vi "Create PVConnections.vi"(8 "error in (no error)":errorcluster, 11 "BNT_ULx-MCSV in":refnum<class "BNT_ULx-MCSV.lvclass">) -> (0 "error out":errorcluster, 3 "BNT_ULx-MCSV out":refnum<class "BNT_ULx-MCSV.lvclass">)   [LabVIEW 2021, in "BNT_ULx.lvlib" / "BNT_ULx-MCSV.lvclass"]
doc: "Create PVConnection objects"
uses:
  BNT_ULx-MCSV.lvclass
  C:/Users/Holger/Documents/LVP/CSPP/CSPP-Template/Packages/CSPP_Core/Actors/CSPP_BaseActor/CSPP_BaseActor.lvclass
  CSPP_Core/Actors/CSPP_BaseActor/CSPP_BaseActor.lvclass/CSPP_BaseActor.ctl
  BNT_ULx-MCSV.lvclass/BNT_ULx-MCSV.ctl
  CSPP_Core/Classes/CSPP_BaseClasses/Factory/CSPP_Factory.lvclass
  CSPP_Core/Actors/CSPP_BaseActor/CSPP_BaseActor.lvclass
  CSPP_Core/Classes/CSPP_ProcessVariables/CSPP_ProcessVariables.lvlib
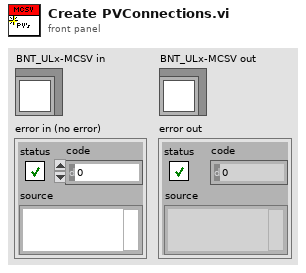
[diagram p1: front panel]
types:
  T1 = cluster{string, "Type Descriptor":string, string}
  T2 = cluster{"initial string":string, "Type Descriptor":string, string}
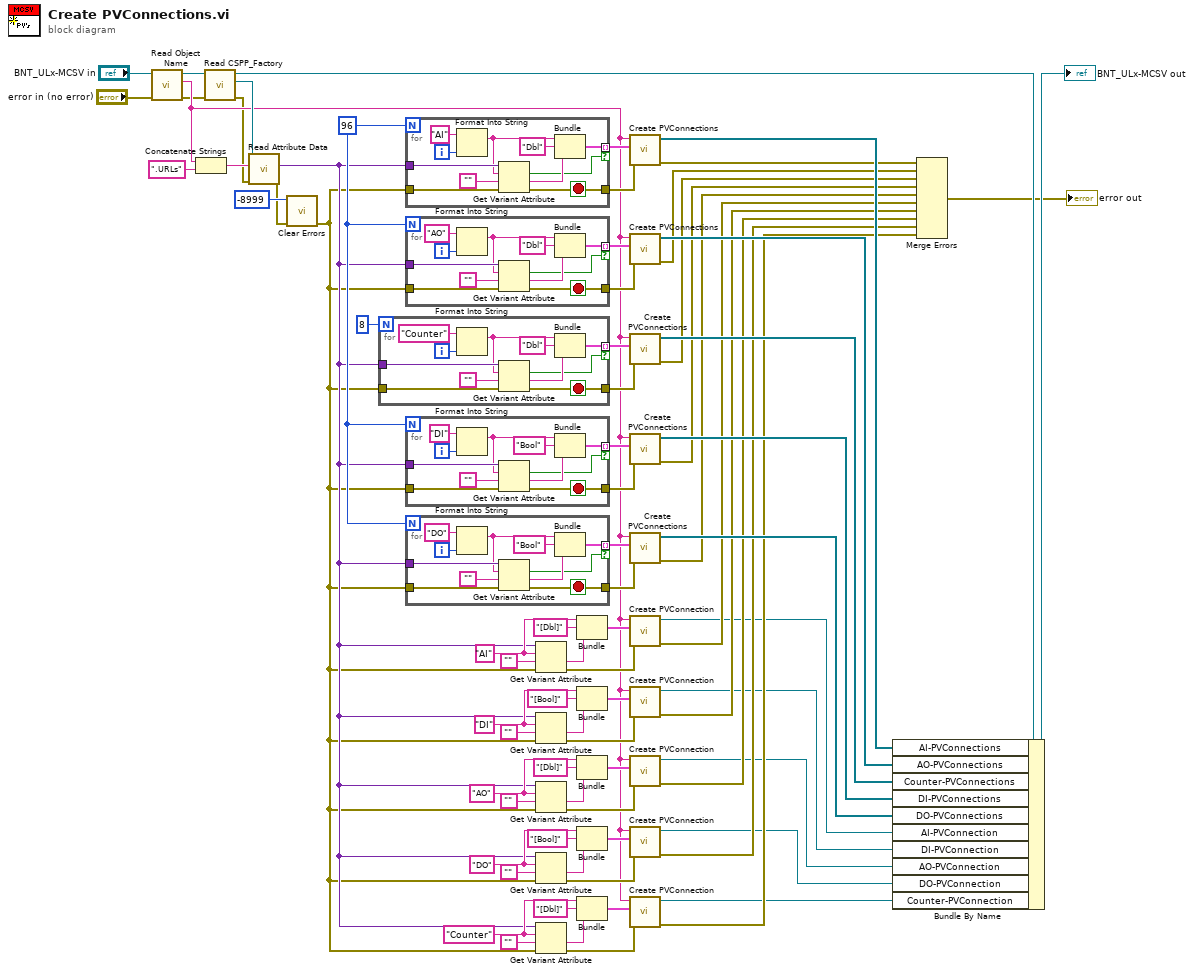
[diagram p0: block diagram]
diagram:
  w20 = "Counter" ("initial string")
  w34 = "DO" ("initial string")
  w27 = "AO" ("initial string")
  w40 = "DI" ("initial string")
  w48 = "AI" ("initial string")
  w52 = 96
  n1 = call "Read Object Name.vi"("error in (no error)"="error in (no error)", "CSPP_BaseActor in"="BNT_ULx-MCSV in") -> ("error out"=w4:errorcluster, "Object Name"=w16:string, "CSPP_BaseActor out"=w78:refnum<class "BNT_ULx-MCSV.lvclass">)  [unwired: 7 in]
  n2 = Concatenate Strings(w16, ".URLs" ("string")) -> (w76:string)
  n3 = call "Read CSPP_Factory.vi"("error in (no error)"=w4, "CSPP_BaseActor in"=w78) -> ("error out"=w3:errorcluster, "CSPP_Factory"=w73:refnum<class "CSPP_Factory.lvclass">, "CSPP_BaseActor out"=w7:refnum<class "BNT_ULx-MCSV.lvclass">)  [unwired: 7 in]
  n4 = call-dynamic "Read Attribute Data.vi"("error in (no error)"=w3, "Object Name"=w76, "CSPP_Factory in"=w73) -> ("error out"=w74:errorcluster, "Attribute Data"=w15:variant)  [unwired: 6 in, 1 out]
  n5 = call <vilib>:"Clear Errors.vi"("error in (no error)"=w74, "specific error code to clear (0: all)"=-8999) -> ("error out"=w14:errorcluster)  [unwired: 4 in, 1 out]
  n6 = for {
    N: 8 -> [_]
    tunnel: w15 -> [w88]
    tunnel: w14 -> [w87]
    tunnel: [w83] -> w63 mode=indexing if=w80
    tunnel: [w79] -> w62
    i -> [w86]
    stop <- w79 stop-if-true
    n7 = Format Into String(initial string="Counter", w86) -> (resulting string=w84:string)  [unwired: 2 in, 1 out]
    n8 = Get Variant Attribute(Variant=w88, name=w84, default value (empty Variant)="", error in=w87) -> (found=w80:bool, value=w81:string, error out=w79:errorcluster)  [unwired: 1 out]
    n9 = Bundle(w84, "Type Descriptor"="Dbl", w81) -> (w83:T1)  [unwired: 1 in]
  }
  n10 = for {
    N: w52 -> [_]
    tunnel: w15 -> [w99]
    tunnel: w14 -> [w98]
    tunnel: [w94] -> w71 mode=indexing if=w91
    tunnel: [w90] -> w68
    i -> [w97]
    stop <- w90 stop-if-true
    n11 = Format Into String(initial string="AI", w97) -> (resulting string=w95:string)  [unwired: 2 in, 1 out]
    n12 = Get Variant Attribute(Variant=w99, name=w95, default value (empty Variant)="", error in=w98) -> (found=w91:bool, value=w92:string, error out=w90:errorcluster)  [unwired: 1 out]
    n13 = Bundle(w95, "Type Descriptor"="Dbl", w92) -> (w94:T1)  [unwired: 1 in]
  }
  n14 = for {
    N: w52 -> [_]
    tunnel: w15 -> [w110]
    tunnel: w14 -> [w109]
    tunnel: [w105] -> w66 mode=indexing if=w102
    tunnel: [w101] -> w67
    i -> [w108]
    stop <- w101 stop-if-true
    n15 = Format Into String(initial string="AO", w108) -> (resulting string=w106:string)  [unwired: 2 in, 1 out]
    n16 = Get Variant Attribute(Variant=w110, name=w106, default value (empty Variant)="", error in=w109) -> (found=w102:bool, value=w103:string, error out=w101:errorcluster)  [unwired: 1 out]
    n17 = Bundle(w106, "Type Descriptor"="Dbl", w103) -> (w105:T1)  [unwired: 1 in]
  }
  n18 = for {
    N: w52 -> [_]
    tunnel: w15 -> [w121]
    tunnel: w14 -> [w120]
    tunnel: [w116] -> w58 mode=indexing if=w113
    tunnel: [w112] -> w57
    i -> [w119]
    stop <- w112 stop-if-true
    n19 = Format Into String(initial string="DI", w119) -> (resulting string=w117:string)  [unwired: 2 in, 1 out]
    n20 = Get Variant Attribute(Variant=w121, name=w117, default value (empty Variant)="", error in=w120) -> (found=w113:bool, value=w114:string, error out=w112:errorcluster)  [unwired: 1 out]
    n21 = Bundle(w117, "Type Descriptor"="Bool", w114) -> (w116:T1)  [unwired: 1 in]
  }
  n22 = for {
    N: w52 -> [_]
    tunnel: w15 -> [w132]
    tunnel: w14 -> [w131]
    tunnel: [w127] -> w53 mode=indexing if=w124
    tunnel: [w123] -> w54
    i -> [w130]
    stop <- w123 stop-if-true
    n23 = Format Into String(initial string="DO", w130) -> (resulting string=w128:string)  [unwired: 2 in, 1 out]
    n24 = Get Variant Attribute(Variant=w132, name=w128, default value (empty Variant)="", error in=w131) -> (found=w124:bool, value=w125:string, error out=w123:errorcluster)  [unwired: 1 out]
    n25 = Bundle(w128, "Type Descriptor"="Bool", w125) -> (w127:T1)  [unwired: 1 in]
  }
  n26 = Get Variant Attribute(Variant=w15, name=w48, default value (empty Variant)="", error in=w14) -> (value=w47:string, error out=w44:errorcluster)  [unwired: 2 out]
  n27 = Get Variant Attribute(Variant=w15, name=w40, default value (empty Variant)="", error in=w14) -> (value=w41:string, error out=w43:errorcluster)  [unwired: 2 out]
  n28 = Get Variant Attribute(Variant=w15, name=w27, default value (empty Variant)="", error in=w14) -> (value=w28:string, error out=w30:errorcluster)  [unwired: 2 out]
  n29 = Get Variant Attribute(Variant=w15, name=w34, default value (empty Variant)="", error in=w14) -> (value=w33:string, error out=w31:errorcluster)  [unwired: 2 out]
  n30 = Get Variant Attribute(Variant=w15, name=w20, default value (empty Variant)="", error in=w14) -> (value=w19:string, error out=w17:errorcluster)  [unwired: 2 out]
  n31 = Bundle("initial string"=w48, "Type Descriptor"="[Dbl]", w47) -> (w46:T2)  [unwired: 1 in]
  n32 = Bundle("initial string"=w40, "Type Descriptor"="[Bool]", w41) -> (w42:T2)  [unwired: 1 in]
  n33 = Bundle("initial string"=w27, "Type Descriptor"="[Dbl]", w28) -> (w29:T2)  [unwired: 1 in]
  n34 = Bundle("initial string"=w34, "Type Descriptor"="[Bool]", w33) -> (w32:T2)  [unwired: 1 in]
  n35 = Bundle("initial string"=w20, "Type Descriptor"="[Dbl]", w19) -> (w18:T2)  [unwired: 1 in]
  n36 = call "Create PVConnections.vi"("Error In"=w68, "PV-Infos"=w71, "Object Name"=w16) -> ("error out"=w69:errorcluster, "PVConnections"=w70:refnum<class "PVConnection.lvclass">[])  [unwired: 7 in]
  n37 = call "Create PVConnections.vi"("Error In"=w67, "PV-Infos"=w66, "Object Name"=w16) -> ("error out"=w64:errorcluster, "PVConnections"=w65:refnum<class "PVConnection.lvclass">[])  [unwired: 7 in]
  n38 = call "Create PVConnections.vi"("Error In"=w62, "PV-Infos"=w63, "Object Name"=w16) -> ("error out"=w59:errorcluster, "PVConnections"=w60:refnum<class "PVConnection.lvclass">[])  [unwired: 7 in]
  n39 = call "Create PVConnections.vi"("Error In"=w57, "PV-Infos"=w58, "Object Name"=w16) -> ("error out"=w55:errorcluster, "PVConnections"=w56:refnum<class "PVConnection.lvclass">[])  [unwired: 7 in]
  n40 = call "Create PVConnections.vi"("Error In"=w54, "PV-Infos"=w53, "Object Name"=w16) -> ("error out"=w50:errorcluster, "PVConnections"=w51:refnum<class "PVConnection.lvclass">[])  [unwired: 7 in]
  n41 = call "Create PVConnection.vi"("Error In"=w44, "PV-Info"=w46, "Object Name"=w16) -> ("error out"=w45:errorcluster, "PVConnection"=w12:refnum<class "PVConnection.lvclass">)  [unwired: 7 in]
  n42 = call "Create PVConnection.vi"("Error In"=w43, "PV-Info"=w42, "Object Name"=w16) -> ("error out"=w37:errorcluster, "PVConnection"=w11:refnum<class "PVConnection.lvclass">)  [unwired: 7 in]
  n43 = call "Create PVConnection.vi"("Error In"=w30, "PV-Info"=w29, "Object Name"=w16) -> ("error out"=w24:errorcluster, "PVConnection"=w10:refnum<class "PVConnection.lvclass">)  [unwired: 7 in]
  n44 = call "Create PVConnection.vi"("Error In"=w31, "PV-Info"=w32, "Object Name"=w16) -> ("error out"=w23:errorcluster, "PVConnection"=w9:refnum<class "PVConnection.lvclass">)  [unwired: 7 in]
  n45 = call "Create PVConnection.vi"("Error In"=w17, "PV-Info"=w18, "Object Name"=w16) -> ("error out"=w13:errorcluster, "PVConnection"=w1:refnum<class "PVConnection.lvclass">)  [unwired: 7 in]
  n46 = Bundle By Name(cluster=w7, "AI-PVConnections"=w70, "AO-PVConnections"=w65, "Counter-PVConnections"=w60, "DI-PVConnections"=w56, "DO-PVConnections"=w51, "AI-PVConnection"=w12, "DI-PVConnection"=w11, "AO-PVConnection"=w10, "DO-PVConnection"=w9, "Counter-PVConnection"=w1) -> (→"BNT_ULx-MCSV out":refnum<class "BNT_ULx-MCSV.lvclass">)
  n47 = Merge Errors(w69, w64, w59, w55, w50, w45, w37, w24, w23, w13) -> (→"error out":errorcluster)
